vi "Update Distance and Angle to Wall Using Lidar Continuously.vi"(11 "OH SHIT, STOP":bool) -> (3 "OH SHIT NO LIDAR DATA!!!":bool)   [LabVIEW 2016]
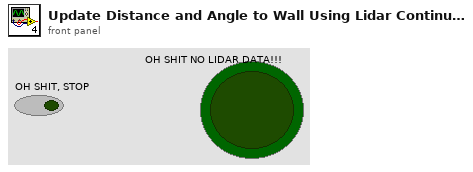
[diagram p1: front panel]
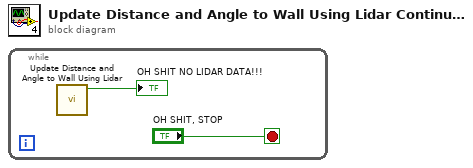
[diagram p0: block diagram]
diagram:
  n1 = while {
    stop <- "OH SHIT, STOP" stop-if-true
    n2 = call "Update Distance and Angle to Wall Using Lidar.vi"() -> ("OH SHIT NO LIDAR DATA!!!"=→"OH SHIT NO LIDAR DATA!!!":bool)  [unwired: 11 in]
  }
